vi "fp5ultrasonic.vi"   [LabVIEW 2016]
uses:
  <vilib>/NXT/Block Support/NXT_OutputPort.ctl
  <vilib>/NXT/Block Support/NXT_InputPort.ctl
  <vilib>/NXT/NXTIO Xnodes/NXTIONodeSubVIs/LEGOResetMotors.vi
  <vilib>/NXT/Dual Mode Library/Sensors/EV3_Ultrasonic_CM.vi
  <vilib>/NXT/Dual Mode Library/Sensors/EV3_Color_Reflect.vi
  <vilib>/NXT/NXTIO Xnodes/NXTIONodeSubVIs/NXTMoveMotors.vi
  <vilib>/NXT/NXTIO Xnodes/NXTIONodeSubVIs/NXTMotorRunDistance.vi
  <vilib>/NXT/NXTIO Xnodes/NXTIONodeSubVIs/NXTStopMotors.vi
  <vilib>/NXT/Dual Mode Library/Sound/PlayAsharp.vi
  <vilib>/NXT/Dual Mode Library/Sound/PlayC.vi
  <vilib>/NXT/Subs/LVHSConnector.ctl
  <vilib>/NXT/NXTIO Xnodes/AddressXNode/NXTIOAddress.xnode
  <vilib>/NXT/NXTIO Xnodes/NXTIOXNode/NXTIO.xnode
  <vilib>/NXT/LegoClasses/BrickReference/BrickReference.lvclass
types:
  T1 = typedef "NXT_OutputPort.ctl" = u8
  T2 = typedef "NXT_InputPort.ctl" = u32
  T3 = typedef "LVHSConnector.ctl" = refnum<class "BrickReference.lvclass">
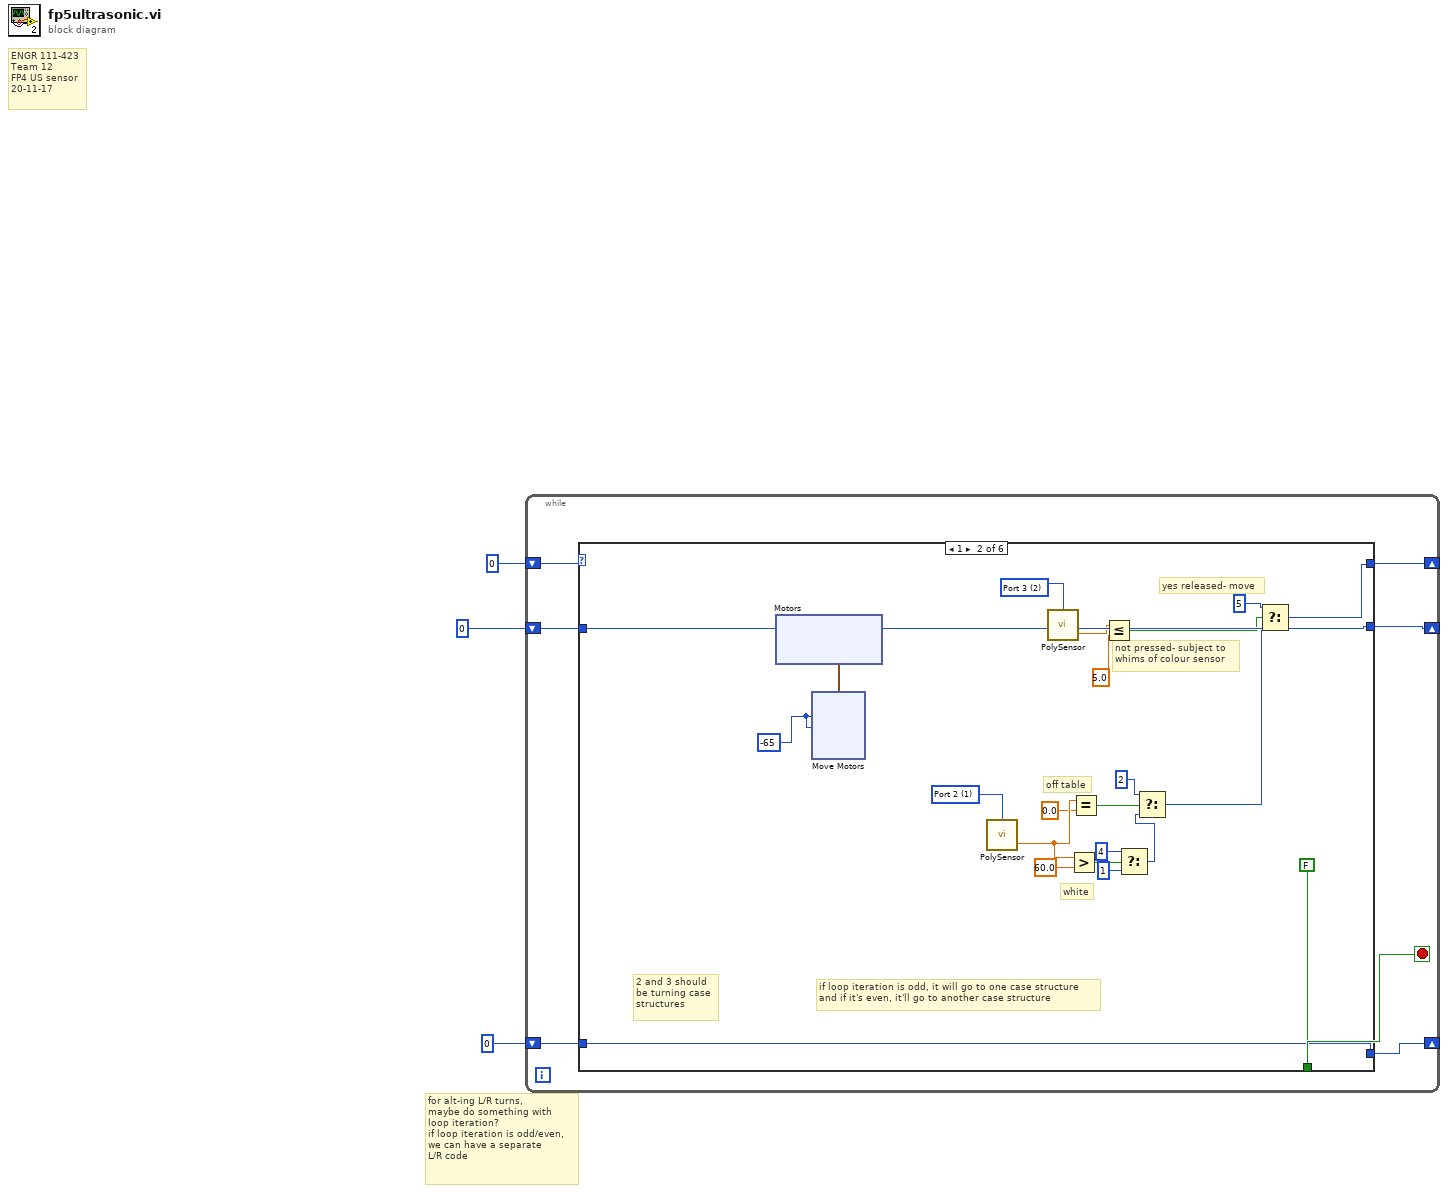
[diagram p0: block diagram]
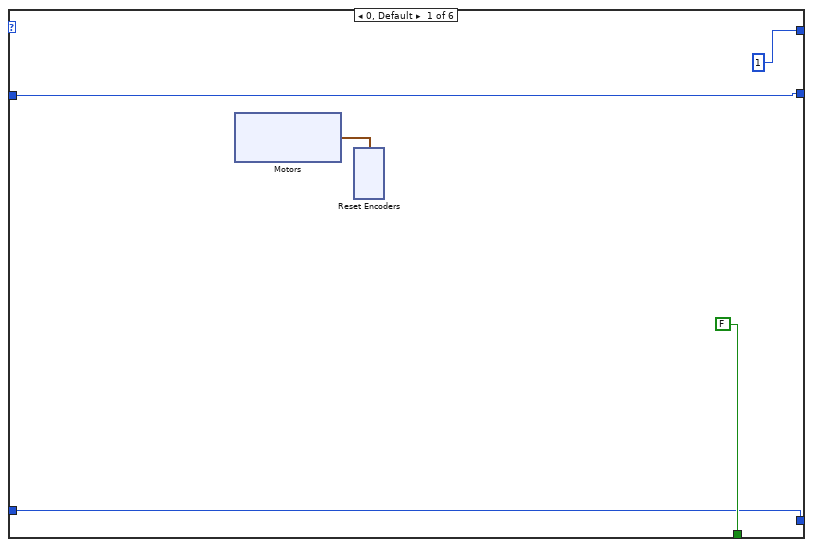
[diagram p2: hidden frame]
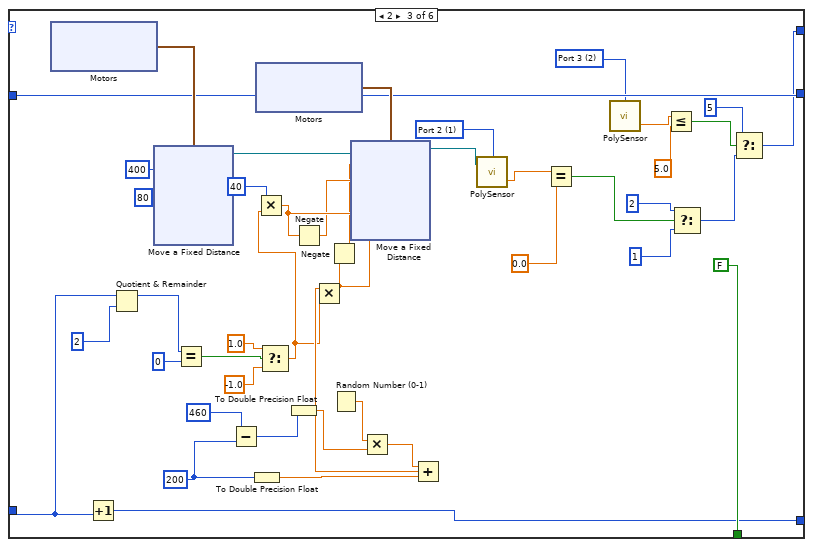
[diagram p3: hidden frame]
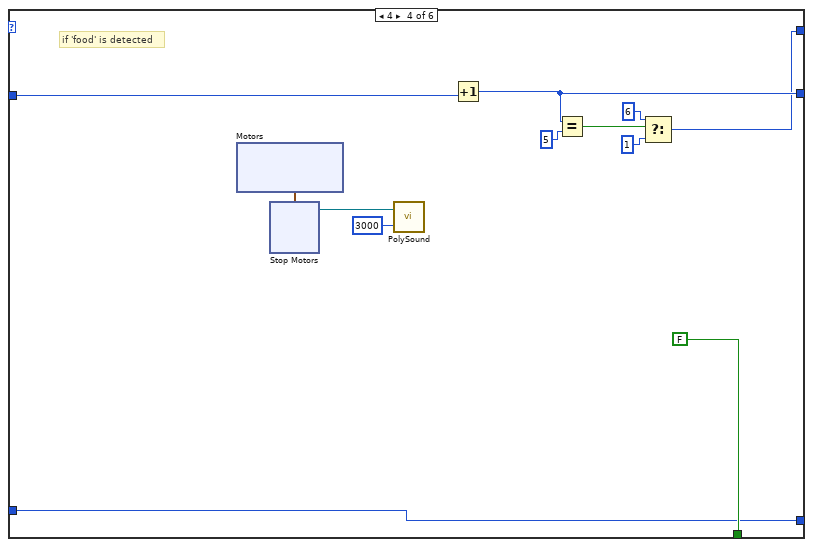
[diagram p4: hidden frame]
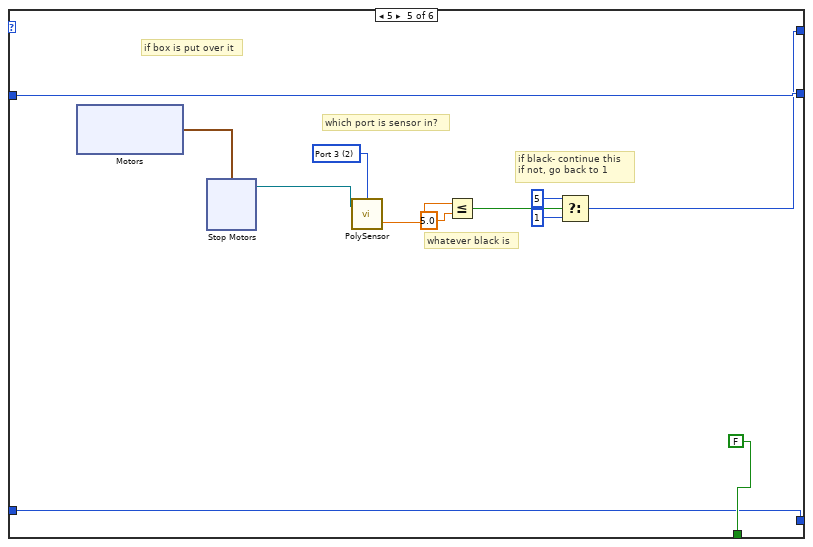
[diagram p5: hidden frame]
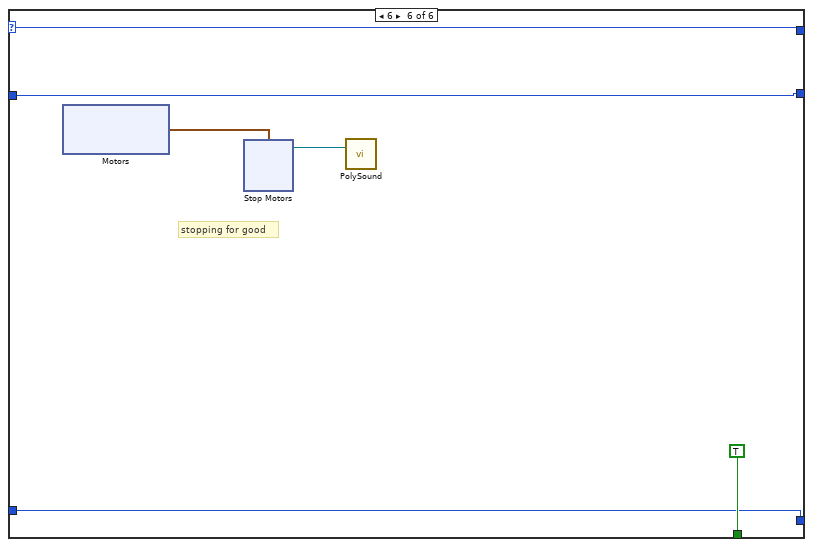
[diagram p6: hidden frame]
diagram:
  # "for alt-ing L/R turns,\nmaybe do something with\nloop iteration?\nif loop iteration is odd/even,\nwe can have a separate\nL/R code"
  # "ENGR 111-423\nTeam 12\nFP4 US sensor\n20-11-17"
  n1 = while {
    shift-right: [w8] -> _
    shift-left: 0 -> [w10]
    shift-right: [w6] -> _
    shift-left: 0 -> [w7]
    shift-right: [w4] -> _
    shift-left: 0 -> [w5]
    stop <- w9 stop-if-true
    n2 = case shown="1" w10 {
      selector: w10 -> [_ _ _ _ _ w161]
      tunnel: [FALSE FALSE FALSE FALSE FALSE TRUE] -> w9
      tunnel: [1 w33 w70 w122 w144 w161] -> w8
      tunnel: w7 -> [w12 w29 w71 w129 w146 w158]
      tunnel: [w12 w29 w71 w126 w146 w158] -> w6
      tunnel: w5 -> [w11 w25 w57 w121 w145 w157]
      tunnel: [w11 w25 w58 w121 w145 w157] -> w4
      frame 0, Default {
        n3 = xnode "Motors"() -> ("Motor"=w13:cluster{"Port":T1, "Port":T1})
        n4 = xnode "Reset Encoders"("Motors"=w13) -> ()  [unwired: 1 in, 1 out]
      }
      frame 1 {
        w34 = T2 1 items=["Port 1", "Port 2", "Port 3", "Port 4"] ("Port (Port 1)")
        w21 = T2 2 items=["Port 1", "Port 2", "Port 3", "Port 4"] ("Port (Port 1)")
        w41 = -65 ("Distance 1")
        # "white"
        # "off table"
        # "2 and 3 should\nbe turning case\nstructures"
        # "if loop iteration is odd, it will go to one case structure\nand if it's even, it'll go to another case structure"
        # "not pressed- subject to\nwhims of colour sensor"
        # "yes released- move"
        n5 = xnode "Motors"() -> ("Motor"=w42:cluster{"Port":T1, "Port":T1})
        n6 = xnode "Move Motors"("Power/Speed 2"=w41, "Power/Speed 1"=w41, "Motors"=w42) -> ()  [unwired: 1 in, 1 out]
        n7 = call-poly <vilib>:"PolySensor.vi"("Port (Port 1)"=w34) -> ("Scaled Value"=w35:sgl)  [unwired: 2 in, 1 out]
        n8 = call-poly <vilib>:"PolySensor.vi"("Port (Port 1)"=w21) -> ("Centimeters"=w24:sgl)  [unwired: 2 in, 1 out]
        n9 = Greater?(x=w35, y=sgl 60.0) -> (0:w39:bool)
        n10 = Equal?(x=w35, y=sgl 0.0) -> (x = y?=w37:bool)
        n11 = Less Or Equal?(x=w24, y=sgl 5.0) -> (x <= y?=w22:bool)
        n12 = Select(t=i16 4, s=w39, f=i16 1) -> (s? t:f=w31:i16)
        n13 = Select(t=2, s=w37, f=w31) -> (s? t:f=w26:i32)
        n14 = Select(t=i16 5, s=w22, f=w26) -> (s? t:f=w33:i32)
      }
      frame 2 {
        w67 = 200
        w84 = 80 ("Distance 1")
        w85 = 400 ("Distance 1")
        w89 = T2 1 items=["Port 1", "Port 2", "Port 3", "Port 4"] ("Port (Port 1)")
        w55 = T2 2 items=["Port 1", "Port 2", "Port 3", "Port 4"] ("Port (Port 1)")
        n15 = xnode "Motors"() -> ("Motor"=w86:cluster{"Port":T1, "Port":T1})
        n16 = Increment(x=w57) -> (x+1=w58:i32)
        n17 = Quotient & Remainder(x=w57, y=2) -> (x-y*floor(x/y)=w78:i32)  [unwired: 1 out]
        n18 = xnode "Move a Fixed Distance"("Speed 2"=w84, "Speed 1"=w84, "Distance 2"=w85, "Distance 1"=w85, "Motors"=w86) -> ("NXT/EV3"=w59:T3)  [unwired: 1 in]
        n19 = Equal?(x=w78, y=0) -> (x = y?=w76:bool)
        n20 = Subtract(x=460, y=w67) -> (x-y=w68:i32)
        n21 = To Double Precision Float(number=w67) -> (double precision float=w63:dbl)
        n22 = xnode "Motors"() -> ("Motor"=w87:cluster{"Port":T1, "Port":T1})
        n23 = Select(t=1.0, s=w76, f=-1.0) -> (s? t:f=w61:dbl)
        n24 = Multiply(x=40 ("Distance 1"), y=w61) -> (x*y=w81:dbl)
        n25 = To Double Precision Float(number=w68) -> (double precision float=w66:dbl)
        n26 = Negate(x=w81) -> (-x=w80:dbl)
        n27 = Random Number (0-1)() -> (number: 0 to 1=w65:dbl)
        n28 = Multiply(x=w65, y=w66) -> (x*y=w64:dbl)
        n29 = Add(x=w64, y=w63) -> (x+y=w62:dbl)
        n30 = Multiply(x=w62, y=w61) -> (x*y=w60:dbl)
        n31 = Negate(x=w60) -> (-x=w73:dbl)
        n32 = xnode "Move a Fixed Distance"("Speed 2"=w81, "Speed 1"=w80, "Distance 2"=w60, "Distance 1"=w73, "Motors"=w87, "NXT/EV3"=w59) -> ("NXT/EV3"=w56:T3)
        n33 = call-poly <vilib>:"PolySensor.vi"("NXT/EV3"=w56, "Port (Port 1)"=w89) -> ("Scaled Value"=w88:sgl)  [unwired: 1 in, 1 out]
        n34 = Equal?(x=w88, y=0.0) -> (x = y?=w90:bool)
        n35 = call-poly <vilib>:"PolySensor.vi"("Port (Port 1)"=w55) -> ("Centimeters"=w54:sgl)  [unwired: 2 in, 1 out]
        n36 = Less Or Equal?(x=w54, y=sgl 5.0) -> (x <= y?=w52:bool)
        n37 = Select(t=2, s=w90, f=1) -> (s? t:f=w93:i32)
        n38 = Select(t=5, s=w52, f=w93) -> (s? t:f=w70:i32)
      }
      frame 4 {
        # "if 'food' is detected"
        n39 = xnode "Motors"() -> ("Motor"=w131:cluster{"Port":T1, "Port":T1})
        n40 = xnode "Stop Motors"("Motors"=w131) -> ("NXT/EV3"=w132:T3)  [unwired: 1 in]
        n41 = call-poly <vilib>:"PolySound.vi"("Duration (500 ms)"=u16 3000, "NXT/EV3"=w132) -> ()  [unwired: 2 in, 1 out]
        n42 = Increment(x=w129) -> (x+1=w126:i32)
        n43 = Equal?(x=w126, y=5) -> (x = y?=w127:bool)
        n44 = Select(t=6, s=w127, f=1) -> (s? t:f=w122:i32)
      }
      frame 5 {
        w142 = T2 2 items=["Port 1", "Port 2", "Port 3", "Port 4"] ("Port (Port 1)")
        # "if black- continue this\nif not, go back to 1"
        # "whatever black is"
        # "which port is sensor in?"
        # "if box is put over it"
        n45 = xnode "Motors"() -> ("Motor"=w150:cluster{"Port":T1, "Port":T1})
        n46 = xnode "Stop Motors"("Motors"=w150) -> ("NXT/EV3"=w143:T3)  [unwired: 1 in]
        n47 = call-poly <vilib>:"PolySensor.vi"("NXT/EV3"=w143, "Port (Port 1)"=w142) -> ("Centimeters"=w141:sgl)  [unwired: 1 in, 1 out]
        n48 = Less Or Equal?(x=w141, y=sgl 5.0) -> (x <= y?=w139:bool)
        n49 = Select(t=i16 5, s=w139, f=i16 1) -> (s? t:f=w144:i16)
      }
      frame 6 {
        # "stopping for good"
        n50 = xnode "Motors"() -> ("Motor"=w162:cluster{"Port":T1, "Port":T1})
        n51 = xnode "Stop Motors"("Motors"=w162) -> ("NXT/EV3"=w159:T3)  [unwired: 1 in]
        n52 = call-poly <vilib>:"PolySound.vi"("NXT/EV3"=w159) -> ()  [unwired: 3 in, 1 out]
      }
    }
  }
